vi "06a-arrays.vi"() -> ()   [LabVIEW 2018, in "LV2Julia_examples.lvlib"]
uses:
  LV2Julia_examples.lvlib
  LV2Julia_core/VIs/Server or client state.ctl
  LV2Julia_core/VIs/detailed error info.ctl
  LV2Julia_core/VIs/StackFrame.ctl
  LV2Julia_core/VIs/Commands.ctl
  72a46192-383e-4ee5-9465-71670922b82a.vi
  ef5408d4-6538-41d1-b296-fda05a71e4b0.vi
  5eac2bf2-d9fb-4bf1-948e-1ebc05516bc9.vi
  e4efb182-1b04-4d49-96a3-1defebd055ea.vi
  ebebf057-8b7e-42d1-8726-0ed76f361650.vi
  72a46192-383e-4ee5-9465-71670922b82a.vi/b0d408ed-daf5-454d-9ecc-f8af6744abda.vi
  ef5408d4-6538-41d1-b296-fda05a71e4b0.vi/f9ecc56d-b53d-412a-9af8-1c97b46c8685.vi
  5eac2bf2-d9fb-4bf1-948e-1ebc05516bc9.vi/6038e038-b9d4-480e-b359-55765becffeb.vi
  e4efb182-1b04-4d49-96a3-1defebd055ea.vi/824be71f-c5ad-4223-87c9-7cdbbdd09736.vi
  e4efb182-1b04-4d49-96a3-1defebd055ea.vi/40be3533-35a9-4e4c-8722-5f4375dd3b08.vi
  e4efb182-1b04-4d49-96a3-1defebd055ea.vi/65a45231-dbbd-4efd-9ebd-6183352d96e2.vi
  e4efb182-1b04-4d49-96a3-1defebd055ea.vi/912004ff-3e56-4cd8-9a85-8f939a39ad48.vi
  ebebf057-8b7e-42d1-8726-0ed76f361650.vi/8b08c596-2b3a-4931-825f-803b1b8d8a5d.vi
  ebebf057-8b7e-42d1-8726-0ed76f361650.vi/babf9289-bc17-4402-9d6c-dd341eb03b80.vi
  ebebf057-8b7e-42d1-8726-0ed76f361650.vi/f5e4d7e9-5b25-498c-b19f-44e63bafc011.vi
  ebebf057-8b7e-42d1-8726-0ed76f361650.vi/f575945d-7167-44e6-afc9-6bef2b394933.vi
  72a46192-383e-4ee5-9465-71670922b82a.vi/b0d408ed-daf5-454d-9ecc-f8af6744abda.vi/a9aded84-fb4c-4b99-9bf2-11a6971dcdab.vi
  ef5408d4-6538-41d1-b296-fda05a71e4b0.vi/f9ecc56d-b53d-412a-9af8-1c97b46c8685.vi/e56f9a54-3a9f-4e68-a3a9-7dfa6a6a4783.vi
  5eac2bf2-d9fb-4bf1-948e-1ebc05516bc9.vi/6038e038-b9d4-480e-b359-55765becffeb.vi/5d76a787-a084-427e-85a3-db925587973b.vi
  5eac2bf2-d9fb-4bf1-948e-1ebc05516bc9.vi/6038e038-b9d4-480e-b359-55765becffeb.vi/e4730504-66cf-4ddf-a61a-738304f2b12e.vi
  5eac2bf2-d9fb-4bf1-948e-1ebc05516bc9.vi/6038e038-b9d4-480e-b359-55765becffeb.vi/49c4ac3b-f14f-40d7-9f02-da6dfb9a79c9.vi
  e4efb182-1b04-4d49-96a3-1defebd055ea.vi/824be71f-c5ad-4223-87c9-7cdbbdd09736.vi/48639029-375b-4425-8f71-319d45f6e3b4.vi
  e4efb182-1b04-4d49-96a3-1defebd055ea.vi/824be71f-c5ad-4223-87c9-7cdbbdd09736.vi/917fea82-d697-4ce0-a076-0fcf05e30575.vi
  <vilib>/Utility/High Resolution Relative Seconds.vi
  ebebf057-8b7e-42d1-8726-0ed76f361650.vi/8b08c596-2b3a-4931-825f-803b1b8d8a5d.vi/7c704175-0edc-4130-a63e-4578cba14c67.vi
  ebebf057-8b7e-42d1-8726-0ed76f361650.vi/8b08c596-2b3a-4931-825f-803b1b8d8a5d.vi/e3978b93-472d-48a9-bab5-51dddfb91b65.vi
  72a46192-383e-4ee5-9465-71670922b82a.vi/b0d408ed-daf5-454d-9ecc-f8af6744abda.vi/a9aded84-fb4c-4b99-9bf2-11a6971dcdab.vi/7b900d93-8f37-40f8-9be1-02a9d42f9a01.vi
  ef5408d4-6538-41d1-b296-fda05a71e4b0.vi/f9ecc56d-b53d-412a-9af8-1c97b46c8685.vi/e56f9a54-3a9f-4e68-a3a9-7dfa6a6a4783.vi/9a698a4f-3967-4c21-99f3-25ec15178b1d.vi
  e4efb182-1b04-4d49-96a3-1defebd055ea.vi/824be71f-c5ad-4223-87c9-7cdbbdd09736.vi/48639029-375b-4425-8f71-319d45f6e3b4.vi/a5759c25-ed5d-4abc-9007-e1bfd2f512dd.vi
  ebebf057-8b7e-42d1-8726-0ed76f361650.vi/8b08c596-2b3a-4931-825f-803b1b8d8a5d.vi/7c704175-0edc-4130-a63e-4578cba14c67.vi/0dcbc56f-df0e-4a08-a62c-191f3a396a75.vi
  LV2Julia_core/VIs/jl-scripts path.vi
  LV2Julia_core/VIs/check ID validity.vi
  LV2Julia_core/VIs/bindata_descr to JSON.vi
  LV2Julia_core/VIs/check cluster field names.vi
  LV2Julia_core/VIs/concat JSON.vi
  LV2Julia_core/VIs/build request.vi
  LV2Julia_core/VIs/Parse server response.vi
  LV2Julia_core/VIs/log jl exceptions.vi
  <vilib>/Utility/error.llb/Error Cluster From Error Code.vi
  LV2Julia_core/LV2Julia_core.lvlib
panel:
  in  "invert matrix":cluster{"invert":bool}={"invert"=TRUE}
  out "inverted matrix":dbl[][](array[numeric])=[[1.0, 0.0, 5.0], [4.0, 2.0, 1.0], [2.0, 2.0, 3.0]] format="%#.4g"
  out "determinant":dbl
  out "Solution Vector":dbl[](array[numeric]) format="%.2f"
  in  "Known Vector":dbl[](array[numeric])=[22.0, 14.0, 18.0]
  in  "Input Matrix":dbl[][](array[numeric])=[[1.0, 0.0, 5.0], [4.0, 2.0, 1.0], [2.0, 2.0, 3.0]]
  in  "next":bool
  out "detailed error info":T1
  out "current error":errorcluster
  out "final error":errorcluster
  out "short err code":u8
  in  "stop":bool
  out "ZMQ timeout":bool
  out "Julia script file path":path
  out "temporary script path":path
  out "Jl Server state":T3
  # "A Bool scalar, a 2D and a 1D array of Float are sent as arguments. \n\nA 1D array and optionally a 2D array and a scalar are returned."
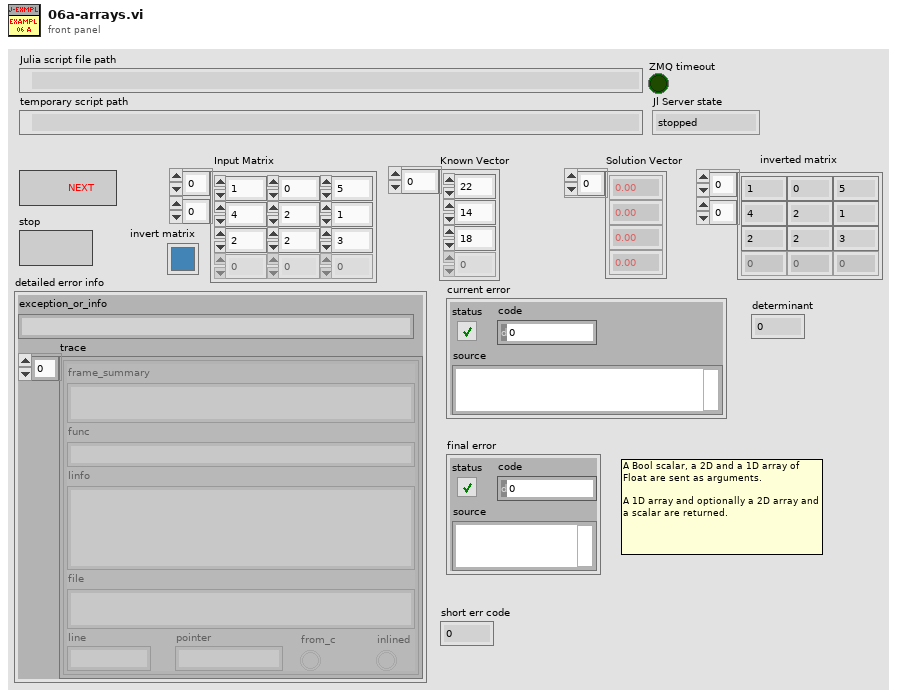
[diagram p1: front panel]
types:
  T1 = typedef "LV2Julia_core.lvlib/detailed error info.ctl" = cluster{"exception_or_info":string, "trace":T2[]}
  T2 = typedef "LV2Julia_core.lvlib/StackFrame.ctl" = cluster{"frame_summary":string, "func":string, "linfo":string, "file":string, "line":i32, "pointer":u64, "from_c":bool, "inlined":bool}
  T3 = typedef "LV2Julia_core.lvlib/Server or client state.ctl" = enum16{"stopped", "running", "unknown"}
  T4 = typedef "LV2Julia_core.lvlib/Commands.ctl" = enum16{"Start Jl-server & Init LV-client", "Send request & Get response ", "Stop Jl-server & Cleanup LV-client", "Cleanup LV-client", "Start Jl-server", "Stop Jl-server", "Init LV-Client", "Cleanup LV-Client", "(not allowed)", "Set LV Client state", "Set Jl Server state", "set ZMQ timeout", "read ZMQ timeout", "read-out state"}
  T5 = typedef "LV2Julia_core.lvlib/Bindata&description.ctl" = cluster{"bindata_descr":T6[], "bindata":u8[]}
  T6 = typedef "LV2Julia_core.lvlib/Bindata description.ctl" = cluster{"nofbytes":i32, "numtype":string, "start":i32, "arrdims":i32[], "kwarg_name":string, "category":string}
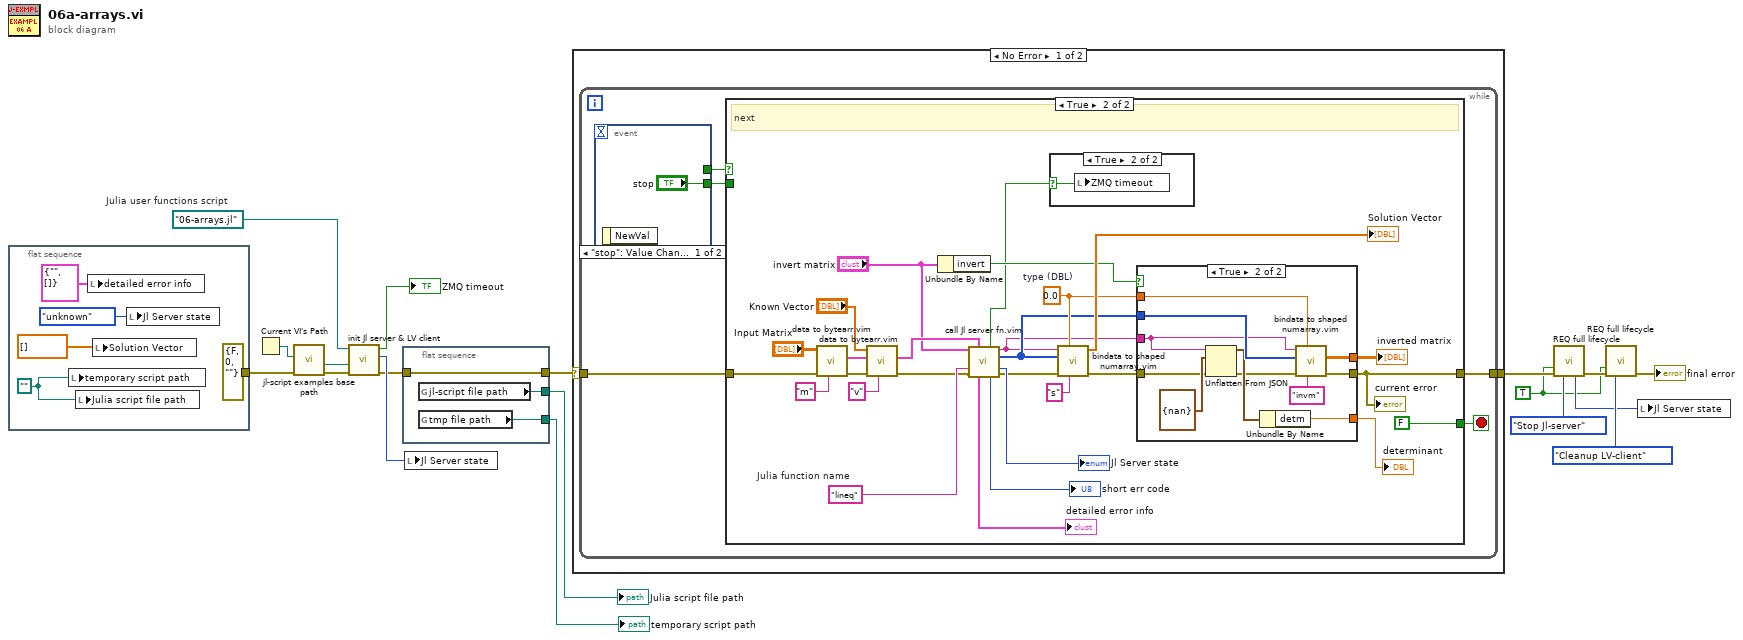
[diagram p0: block diagram]
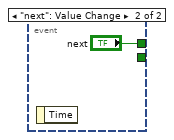
[diagram p2: hidden frame]
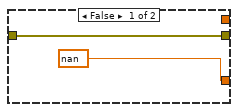
[diagram p4: hidden frame]
diagram:
  w8 = path "06-arrays.jl"  # Julia user functions script
  w9 = TRUE ("Force command")
  n1 = flat-sequence {
    tunnel: [errorcluster {"status"=FALSE, "code"=0, "source"=""} ("error in (no error)")] -> w1
    frame #0 {
      w19 = path ""
      n2 = local write "temporary script path"(w19) -> ()
      n3 = local write "Julia script file path"(w19) -> ()
      n4 = local write "detailed error info"(T1 {"exception_or_info"="", "trace"=[]} ("detailed error info")) -> ()
      n5 = local write "Solution Vector"(dbl[] [] ("Server response")) -> ()
      n6 = local write "Jl Server state"(Server_or_client_state."unknown" ("Jl Server state out")) -> ()
    }
  }
  n7 = Current VI's Path() -> (path=w4:path)
  n8 = call "jl-script examples base path.vi"("error in (no error)"=w1, "calling example VI path"=w4) -> ("error out"=w3:errorcluster, "jl-script-examples base path"=w2:path)  [unwired: 8 in]
  n9 = call "init Jl server & LV client.vi"("error in (no error)"=w3, "Base path (not a path)"=w2, "Julia user functions script"=w8) -> ("error out"=w5:errorcluster, "Jl Server state out"=w6:T3, "timeout?"=→"ZMQ timeout":bool)  [unwired: 6 in]
  n10 = flat-sequence {
    tunnel: [w26] -> w13
    tunnel: w5 -> [w26]
    tunnel: [w25] -> w11
    tunnel: [w24] -> w12
    frame #0 {
      n11 = global read "jl-scripts path.vi" "jl-script file path"() -> (w25:path)
      n12 = global read "jl-scripts path.vi" "tmp file path"() -> (w24:path)
    }
  }
  n13 = local write "Jl Server state"(w6) -> ()
  n14 = case shown="No Error" w13 {
    selector: w13 -> [w27 w79]
    tunnel: [w28 w79] -> w18
    frame No Error {
      n15 = while {
        tunnel: w27 -> [w32]
        tunnel: [w33] -> w28
        stop <- w30 stop-if-true
        n16 = event shown="[0] \"stop\": Value Change" {
          selector: _ -> [_ _]
          dyn-events: _ -> [_ _]
          timeout: _ -> [_ _]
          tunnel: [_ "next"] -> w31
          tunnel: ["stop" _] -> w29
          event "stop": Value Change {
            n17 = event-data() -> ()  [unwired: 1 in, 1 out]
          }
          event "next": Value Change {
            n18 = event-data() -> ()  [unwired: 1 in, 1 out]
          }
        }
        n19 = case shown="True" w31 {
          tunnel: [w37 w44] -> w33
          tunnel: w32 -> [w37 w59]
          tunnel: [w36 FALSE ("stop this VI only")] -> w30
          tunnel: w29 -> [w36 _]
          frame False {
            # "stop"
          }
          frame True {
            w54 = 0.0  # type (DBL)
            w48 = "lineq"  # Julia function name
            # "next"
            n20 = call "data to bytearr.vim"("kwarg_name"="m", "error in (no error)"=w59, "data in"="Input Matrix") -> ("error out"=w62:errorcluster, "Bindata & descr out"=w61:T5)  [unwired: 6 in, 1 out]
            n21 = call "data to bytearr.vim"("kwarg_name"="v", "error in (no error)"=w62, "Bindata & descr in"=w61, "data in"="Known Vector") -> ("error out"=w47:errorcluster, "Bindata & descr out"=w46:T5)  [unwired: 5 in, 1 out]
            n22 = Unbundle By Name("invert matrix") -> ("invert"=w42:bool)
            n23 = call "call Jl server fn.vim"("Arguments 1"="invert matrix", "Bindata & descr in"=w46, "fun2call"=w48, "error in (no error)"=w47) -> ("timeout?"=w41:bool, "JSON received"=w40:string, "binary data received"=w45:u8[], "Jl Server state out"=→"Jl Server state":T3, "detailed error info"=→"detailed error info":T1, "return code"=→"short err code":u8, "error out"=w49:errorcluster)  [unwired: 5 in]
            n24 = case shown="True" w41 {
              selector: w41 -> [_ w78]
              frame False {
              }
              frame True {
                n25 = local write "ZMQ timeout"(w78) -> ()
              }
            }
            n26 = call "bindata to shaped numarray.vim"("name"="s" ("kwarg_name"), "element type"=w54, "error in (no error)"=w49, "binary data"=w45, "JSON in"=w40) -> ("error out"=w39:errorcluster, "numarray 1D"=→"Solution Vector":dbl[])  [unwired: 1 in, 4 out]
            n27 = case shown="True" w42 {
              tunnel: w54 -> [_ w76]
              tunnel: [_ w75] -> w53
              tunnel: w45 -> [_ w74]
              tunnel: w40 -> [_ w68]
              tunnel: [w66 w73] -> w44
              tunnel: w39 -> [w66 w71]
              tunnel: [nan ("detm") w67] -> w38
              frame False {
              }
              frame True {
                n28 = Unflatten From JSON(JSON string=w68, type and defaults=cluster{"detm":dbl} {"detm"=nan}, error in (no error)=w71) -> (value=w70:cluster{"detm":dbl}, error out=w69:errorcluster)  [unwired: 4 in]
                n29 = Unbundle By Name(w70) -> ("detm"=w67:dbl)
                n30 = call "bindata to shaped numarray.vim"("name"="invm" ("kwarg_name"), "element type"=w76, "error in (no error)"=w69, "binary data"=w74, "JSON in"=w68) -> ("error out"=w73:errorcluster, "numarray 2D"=w75:dbl[][])  [unwired: 1 in, 4 out]
              }
            }
            "current error" <- w44
            "inverted matrix" <- w53
            "determinant" <- w38
          }
        }
      }
    }
    frame Error {
    }
  }
  n31 = call "REQ full lifecycle.vi"("Force command"=w9, "error in"=w18, "command"=Commands."Stop Jl-server") -> ("Jl Server state out"=w10:T3, "error out"=w16:errorcluster)  [unwired: 6 in, 5 out]
  n32 = call "REQ full lifecycle.vi"("Force command"=w9, "error in"=w16, "command"=Commands."Cleanup LV-client") -> ("error out"=→"final error":errorcluster)  [unwired: 6 in, 6 out]
  n33 = local write "Jl Server state"(w10) -> ()
  "temporary script path" <- w12
  "Julia script file path" <- w11
